vi "FourFlippingCoins.vi"() -> ()   [LabVIEW 2014]
panel:
  out "Histogram":dynamicdata(graph)
  out "Array":dbl[](array[numeric])
  in  "Number of Trials":dbl
  out "Number of Heads":dbl
  out "Coin 4":bool
  out "Coin 3":bool
  out "Coin 2":bool
  out "Coin 1":bool
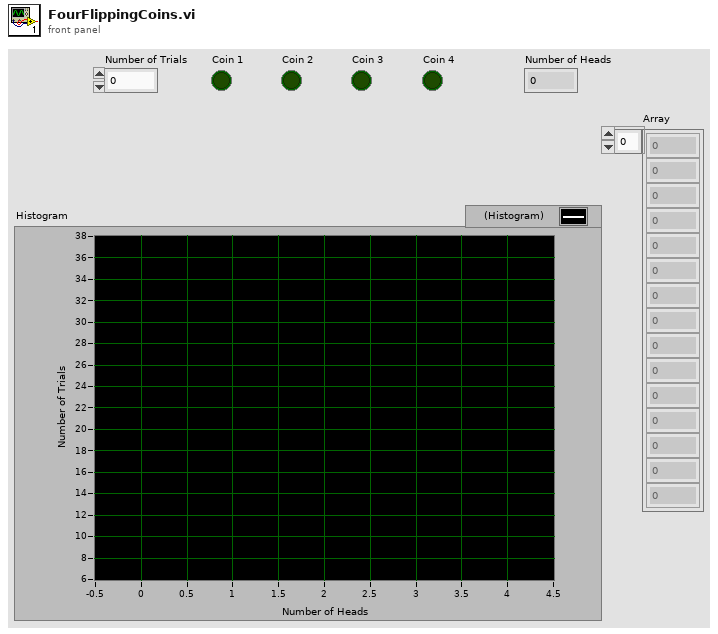
[diagram p1: front panel]
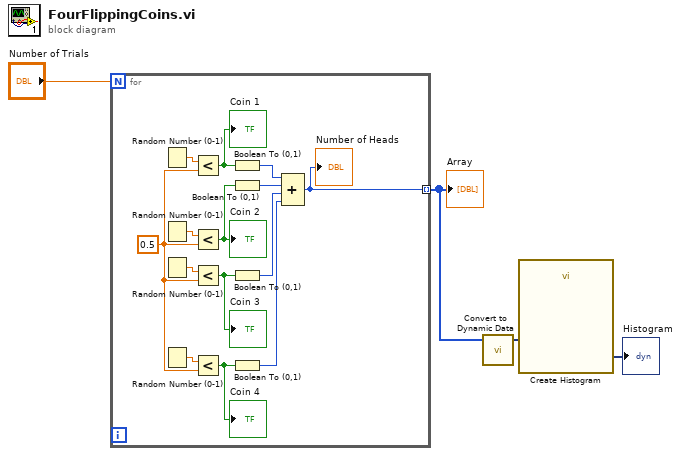
[diagram p0: block diagram]
diagram:
  n1 = for {
    N: "Number of Trials" -> [_]
    tunnel: [w5] -> w3 mode=indexing
    w15 = 0.5
    n2 = Random Number (0-1)() -> (number: 0 to 1=w14:dbl)
    n3 = Random Number (0-1)() -> (number: 0 to 1=w16:dbl)
    n4 = Random Number (0-1)() -> (number: 0 to 1=w18:dbl)
    n5 = Random Number (0-1)() -> (number: 0 to 1=w17:dbl)
    n6 = Less?(x=w14, y=w15) -> (x < y?=w12:bool)
    "Coin 1" <- w12
    n7 = Less?(x=w16, y=w15) -> (x < y?=w8:bool)
    "Coin 2" <- w8
    n8 = Less?(x=w18, y=w15) -> (x < y?=w7:bool)
    "Coin 3" <- w7
    n9 = Less?(x=w17, y=w15) -> (x < y?=w6:bool)
    "Coin 4" <- w6
    n10 = Boolean To (0,1)(Boolean=w12) -> (0, 1=w13:i16)
    n11 = Boolean To (0,1)(Boolean=w8) -> (0, 1=w11:i16)
    n12 = Boolean To (0,1)(Boolean=w7) -> (0, 1=w10:i16)
    n13 = Boolean To (0,1)(Boolean=w6) -> (0, 1=w9:i16)
    n14 = Compound Arithmetic op=ADD(w13, w11, w10, w9) -> (w5:i16)
    "Number of Heads" <- w5
  }
  "Array" <- w3
  n15 = call "Convert to Dynamic Data"("Array"=w3) -> ("Dynamic Data Type"=w2:dynamicdata)  [unwired: 3 in]
  n16 = call "Create Histogram"("Signal"=w2) -> ("Histogram"=→"Histogram":dynamicdata)  [unwired: 9 in, 1 out]
